vi "Test Stop.vi"(0 "VISA resource name":refnum<visa-resource-name>, 11 "error in (no error)":errorcluster) -> (4 "VISA resource name out":refnum<visa-resource-name>, 15 "error out":errorcluster)   [LabVIEW 2016, in "APT 300XAC Series.lvlib"]
doc: "Stops (Power Output Off) the instrument during the test process."
uses:
  APT 300XAC Series.lvlib
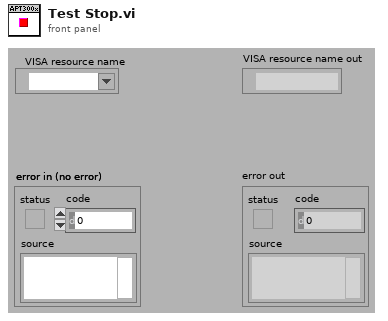
[diagram p1: front panel]
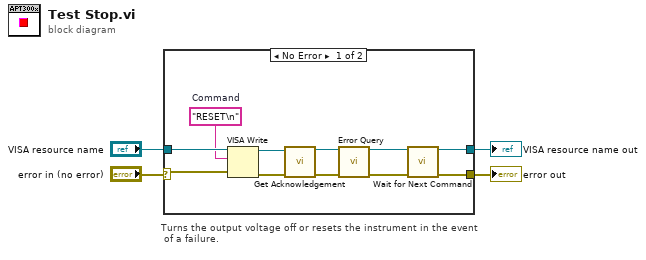
[diagram p0: block diagram]
diagram:
  # "Turns the output voltage off or resets the instrument in the event\n of a failure."
  n1 = case shown="No Error" "error in (no error)" {
    selector: "error in (no error)" -> [w14 w17]
    tunnel: "VISA resource name" -> [w15 w16]
    tunnel: [w7 w16] -> w3
    tunnel: [w8 w17] -> w2
    frame No Error {
      w13 = "RESET\n"  # Command
      n2 = VISA Write(VISA resource name=w15, write buffer=w13, error in (no error)=w14) -> (VISA resource name out=w12:refnum<visa-resource-name>, error out=w11:errorcluster)  [unwired: 1 out]
      n3 = call "Get Acknowledgement.vi"("VISA resource name"=w12, "error in (no error)"=w11) -> ("VISA resource name out"=w10:refnum<visa-resource-name>, "error out"=w9:errorcluster)  [unwired: 12 in]
      n4 = call "Error Query.vi"("VISA resource name"=w10, "error in (no error)"=w9) -> ("VISA resource name out"=w6:refnum<visa-resource-name>, "error out"=w5:errorcluster)  [unwired: 10 in, 2 out]
      n5 = call "Wait for Next Command.vi"("VISA resource name"=w6, "error in (no error)"=w5) -> ("VISA resource name out"=w7:refnum<visa-resource-name>, "error out"=w8:errorcluster)  [unwired: 12 in]
    }
    frame Error {
    }
  }
  "error out" <- w2
  "VISA resource name out" <- w3
